vi "dvr_fgv_map_read.vi"(8 "error in (no error)":errorcluster) -> (0 "error out":errorcluster, 3 "value 2":variant)   [LabVIEW 2020]
uses:
  map_state.ctl
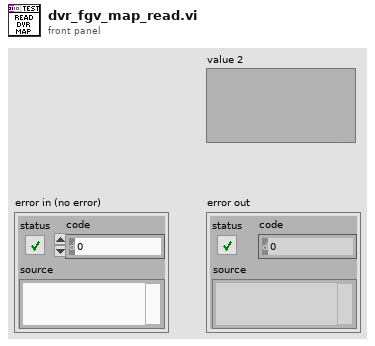
[diagram p1: front panel]
types:
  T1 = typedef "map_state.ctl" = enum16{"flag"}
  T2 = typedef "ram_state.ctl" = enum16{"flag"}
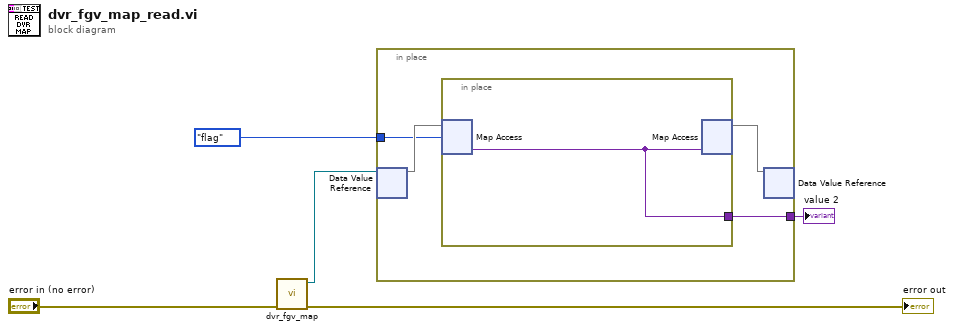
[diagram p0: block diagram]
diagram:
  n1 = call "dvr_fgv_map.vi"("error in (no error)"="error in (no error)") -> ("error out"=→"error out":errorcluster, "data value reference"=w3:refnum<data-value>)  [unwired: 9 in]
  n2 = in-place {
    in-place-border: map_state."flag" ("key") -> [w8]
    in-place-border: [w6] -> w1
    n3 = in-place-dvr #1(w3) -> (w9:map{T2, variant})  [unwired: 1 out]
    n4 = in-place {
      in-place-border: [w10] -> w6
      n5 = in-place-map #2(w9, w8) -> (w10:variant)  [unwired: 1 in, 1 out]
      n6 = in-place-map #2(w10) -> (w7:map{T2, variant})  [unwired: 1 in, 2 out]
    }
    n7 = in-place-dvr #1(w7) -> ()  [unwired: 2 out]
  }
  "value 2" <- w1
